vi "WPI_CameraSend Images to PC Loop_EDIT.vi"(8 "error in (no error)":errorcluster, 9 "port":u16, 10 "Image Name":string, 11 "CameraDevRef":T1) -> ()   [LabVIEW 2015]
doc: "This VI is used to send images to the dashboard using the second enet port on the 8 slot controller. This is provided for compatibility, but is higher overhead than using the Camera MJPG approach.\n\nThis software is licensed. Open the labview\\readme\\WPI Robotics Library Open Source License.txt file for more information."
uses:
  <vilib>/Rock Robotics/WPI/Camera/WPI_CameraDevRef.ctl
  <vilib>/Rock Robotics/SystemInterfaces/NetworkCommunication/NetComm_UsageReport_ResourceType.ctl
  <vilib>/Rock Robotics/Network Tables/NT Read Boolean.vi
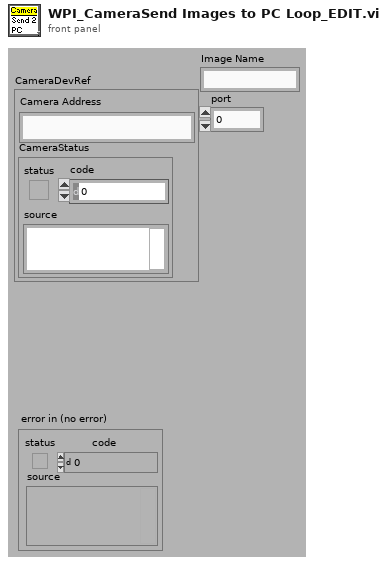
[diagram p1: front panel]
types:
  T1 = typedef "WPI_CameraDevRef.ctl" = cluster{"Camera Address":string, "CameraStatus":errorcluster}
  T2 = cluster{"fps":i32, "compression":i32, "compression 2":i32}
  T3 = typedef "NetComm_UsageReport_ResourceType.ctl" = enum8{"Controller", "Module", "Language", "CANPlugin", "Accelerometer", "ADXL345", "AnalogChannel", "AnalogTrigger", "AnalogTriggerOutput", "CANJaguar", "Compressor", "Counter", "Dashboard", "DigitalInput", "DigitalOutput", "DriverStationCIO", "DriverStationEIO", "DriverStationLCD", "Encoder", "GearTooth", "Gyro", "I2C", "Framework", "Jaguar", "Joystick", "Kinect", "KinectStick", "PIDController", "Preferences", "PWM", "Relay", "RobotDrive", "SerialPort", "Servo", "Solenoid", "SPI", "Task", "Ultrasonic", "Victor", "Button", "Command", "AxisCamera", "PCVideoServer", "SmartDashboard", "Talon", "HiTechnicColorSensor", "HiTechnicAccel", "HiTechnicCompass", "SRF08", "AnalogOutput", "Victor SP", "Talon SRX", "CAN Talon SRX", "ADXL362 Accel", "ADXRS450 Gyro", "Rev SPARK", "Mindsensors SD540", "Digital Filter"}
  T4 = enum16{"Update Mode", "Get Image", "Get Image Data"}
  T5 = typedef "Image Type" = u32
  T6 = typedef "IMAQ Image.ctl" = refnum<image>
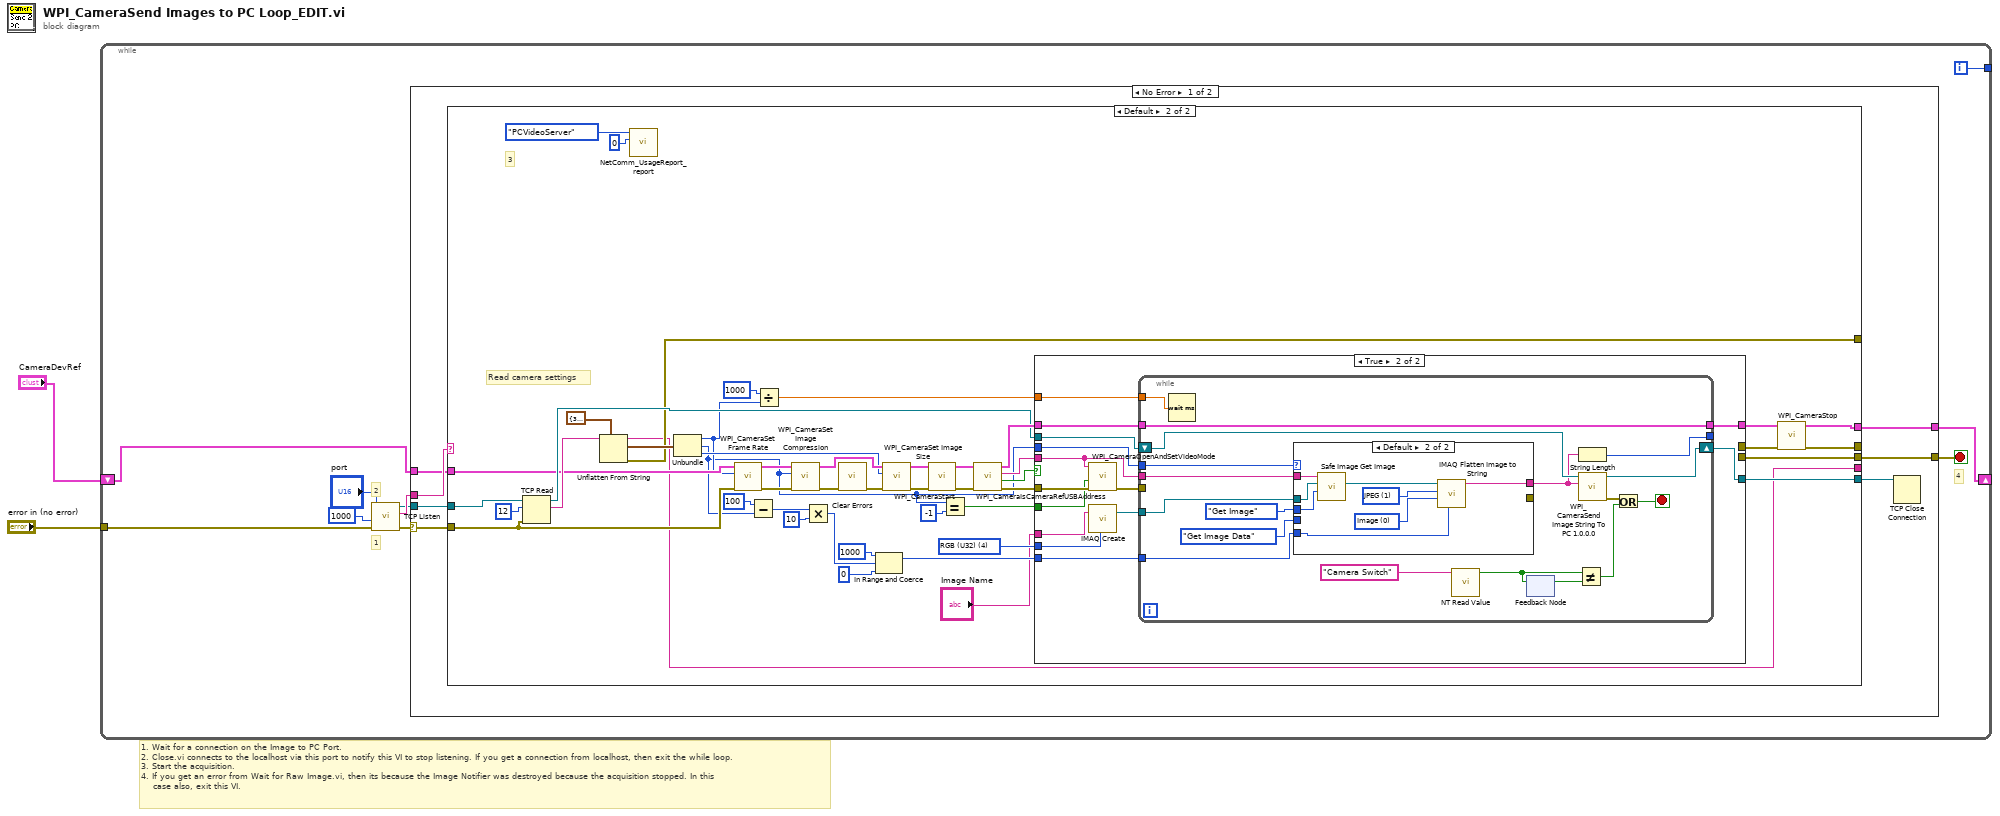
[diagram p0: block diagram]
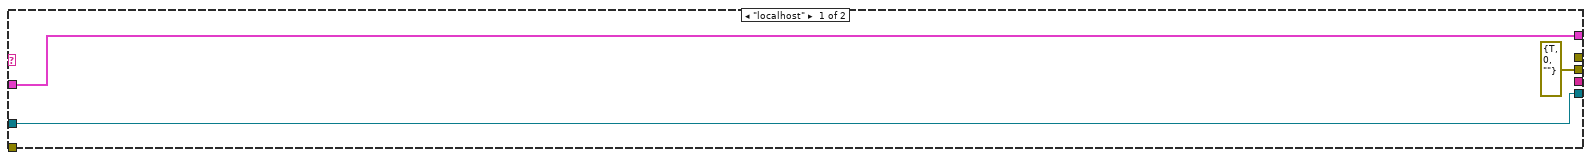
[diagram p2: hidden frame]
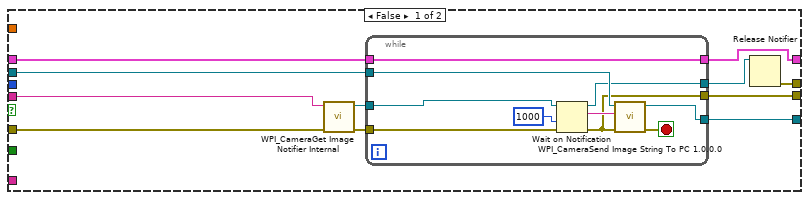
[diagram p3: hidden frame]
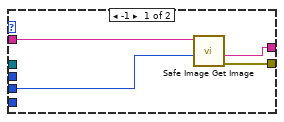
[diagram p4: hidden frame]
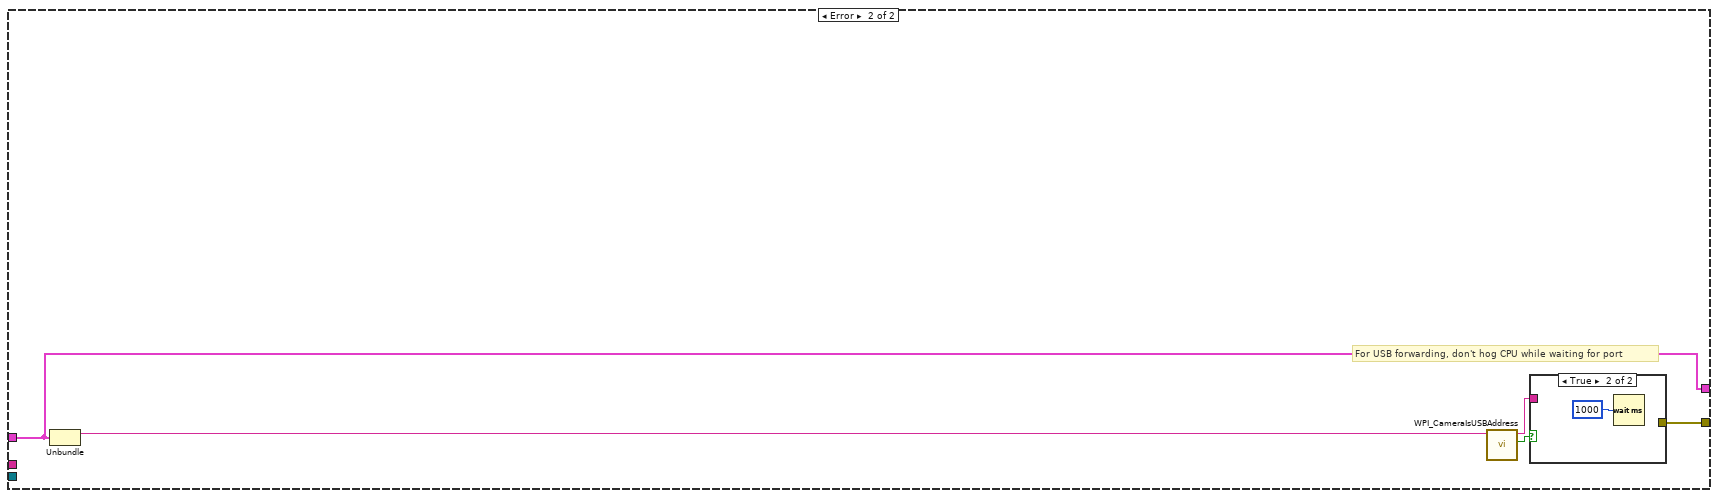
[diagram p5: hidden frame]
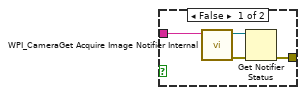
[diagram p6: hidden frame]
diagram:
  # "1. Wait for a connection on the Image to PC Port.\n2. Close.vi connects to the localhost via this port to notify this VI to stop listening. If you get a connection from localhost, then exit the while loop.\n3. Start the acquisition.\n4. If you get an error from Wait for Raw Image.vi, then its because the Image Notifier was destroyed because the acquisition stopped. In this\n    case also, exit this VI."
  n1 = while {
    tunnel: "error in (no error)" -> [w10]
    shift-right: [w12] -> _
    shift-left: "CameraDevRef" -> [w4]
    tunnel: [w5] -> _
    i -> [w5]
    stop <- w8 stop-if-true
    # "4"
    # "1"
    # "2"
    n2 = call <vilib>:"TCP Listen.vi"("error in (no error)"=w10, "timeout ms (wait forever: -1)"=u16 1000 ("port"), "port"="port") -> ("error out"=w7:errorcluster, "remote address"=w11:string, "connection ID"=w9:refnum<k5>)  [unwired: 1 in, 5 out]
    n3 = case shown="No Error" w7 {
      selector: w7 -> [w13 _]
      tunnel: [w19 w138] -> w12
      tunnel: w11 -> [w18 _]
      tunnel: w4 -> [w17 w138]
      tunnel: w9 -> [w16 _]
      tunnel: [w15 w139] -> w8
      frame No Error {
        n4 = case shown="Default" w18 {
          tunnel: [w22 w67] -> w19
          tunnel: w17 -> [w22 w50]
          tunnel: w13 -> [_ w46]
          tunnel: w16 -> [w20 w54]
          tunnel: [errorcluster {"status"=TRUE, "code"=0, "source"=""} ("error out 2") w69] -> w15
          tunnel: [w20 w68] -> w14
          tunnel: [_ w66] -> _
          tunnel: [_ w25] -> _
          tunnel: [_ w24] -> _
          frame "localhost" {
          }
          frame Default {
            w61 = T5 4 items=["Grayscale (U8)", "Grayscale (I16)", "Grayscale (SGL)", "Complex (CSG)", "RGB (U32)", "HSL (U32)", "RGB (U64)", "Grayscale (U16)"] ("Image Type")
            # "Read camera settings"
            # "3"
            n5 = TCP Read(connection ID=w54, bytes to read=12, error in (no error)=w46) -> (connection ID out=w53:refnum<k5>, data out=w51:string)  [unwired: 2 in, 1 out]
            n6 = Unflatten From String(type=T2 {"fps"=30, "compression"=32, "compression 2"=32} ("Camera Settings"), binary string=w51) -> (rest of the binary string=w24:string, value=w43:T2, error out=w25:errorcluster)  [unwired: 3 in]
            n7 = call <vilib>:"NetComm_UsageReport_report.vi"("Instance Number"=u8 0, "Resource Type"=NetComm_UsageReport_ResourceType."PCVideoServer") -> ()  [unwired: 10 in]
            n8 = Unbundle(w43) -> ("fps"=w40:i32, "compression"=w29:i32, "compression 2"=w42:i32)
            n9 = call <vilib>:"WPI_CameraSet Frame Rate.vi"("error in (no error)"=w46, "Frame Rate (fps)"=w40, "CameraDevRef"=w50) -> ("error out"=w45:errorcluster, "CameraDevRef Out"=w49:T1)  [unwired: 7 in]
            n10 = Subtract(x=100, y=w29) -> (x-y=w34:i32)
            n11 = Divide(x=u16 1000 ("port"), y=w40) -> (x/y=w39:dbl)
            n12 = call <vilib>:"WPI_CameraSet Image Compression.vi"("error in (no error)"=w45, "Compression"=w29, "CameraDevRef"=w49) -> ("error out"=w27:errorcluster, "CameraDevRef Out"=w48:T1)  [unwired: 7 in]
            n13 = Multiply(x=w34, y=10) -> (x*y=w36:i32)
            n14 = call <vilib>:"Clear Errors.vi"("error in (no error)"=w27) -> ("error out"=w26:errorcluster)  [unwired: 5 in, 1 out]
            n15 = In Range and Coerce(upper limit=1000, x=w36, lower limit=0) -> (coerced(x)=w32:i32)  [unwired: 1 out]
            n16 = call <vilib>:"WPI_CameraSet Image Size.vi"("error in (no error)"=w26, "Image Size"=w42, "CameraDevRef"=w48) -> ("error out"=w44:errorcluster, "CameraDevRef Out"=w47:T1)  [unwired: 7 in]
            n17 = call <vilib>:"WPI_CameraStart.vi"("error in (no error)"=w44, "CameraDevRef"=w47) -> ("error out"=w58:errorcluster, "CameraDevRef"=w56:T1)  [unwired: 8 out]
            n18 = Equal?(x=w29, y=-1) -> (x = y?=w28:bool)
            n19 = call <vilib>:"WPI_CameraIsCameraRefUSBAddress.vi"("error in (no error)"=w58, "CameraDevRef"=w56) -> ("error out"=w57:errorcluster, "USB?"=w59:bool, "Camera Address Out"=w60:string, "CameraDevRef out"=w55:T1)  [unwired: 6 in]
            n20 = case shown="True" w59 {
              tunnel: w53 -> [w80 w104]
              tunnel: [w79 _] -> w69
              tunnel: [w78 w103] -> w68
              tunnel: w57 -> [w77 w95]
              tunnel: w60 -> [w75 w94]
              tunnel: [w74 w99] -> w65
              tunnel: w55 -> [w73 w100]
              tunnel: [w71 _] -> w64
              tunnel: w61 -> [_ w101]
              tunnel: w32 -> [_ w98]
              tunnel: w39 -> [_ w97]
              tunnel: w29 -> [_ w96]
              tunnel: w28 -> [_ w92]
              tunnel: "Image Name" -> [_ w91]
              frame False {
                n21 = call <vilib>:"WPI_CameraGet Image Notifier Internal.vi"("error in (no error)"=w77, "Camera Address"=w75) -> ("error out"=w76:errorcluster, "Image Notifier"=w72:refnum<notifier>)  [unwired: 8 out]
                n22 = while {
                  tunnel: w76 -> [w86]
                  tunnel: w80 -> [w90]
                  tunnel: [w83] -> w79
                  tunnel: [w88] -> w78
                  tunnel: [w87] -> w74
                  tunnel: w73 -> [w87]
                  tunnel: w72 -> [w85]
                  tunnel: [w81] -> w70
                  stop <- w89 stop-if-true
                  n23 = Wait on Notification(notifier=w85, timeout in ms (-1)=1000 ("Timeout in ms (-1)"), error in (no error)=w86) -> (notifier out=w81:refnum<notifier>, notification=w84:string, error out=w83:errorcluster)  [unwired: 2 out]
                  n24 = call <vilib>:"WPI_CameraSend Image String To PC 1.0.0.0.vi"("error in (no error)"=w83, "String"=w84, "TCP Connection ID"=w90) -> ("error out"=w89:errorcluster, "TCP Connection ID out"=w88:refnum<k5>)  [unwired: 7 out]
                }
                n25 = Release Notifier(notifier=w70) -> (error out=w71:errorcluster)  [unwired: 1 in, 3 out]
              }
              frame True {
                n26 = call <vilib>:"WPI_CameraOpenAndSetVideoMode.vi"("error in (no error)"=w95, "USB JPEG"=w92, "Camera Address Out"=w94) -> ("error out"=w93:errorcluster)  [unwired: 8 in]
                n27 = call "IMAQ Create"("Image Name"=w91, "Image Type"=w101) -> ("New Image"=w102:T6)  [unwired: 3 in, 1 out]
                n28 = while {
                  tunnel: w94 -> [w121]
                  shift-right: [w122] -> w103
                  shift-left: w104 -> [w116]
                  tunnel: w102 -> [w120]
                  tunnel: [w119] -> w99
                  tunnel: w100 -> [w119]
                  tunnel: w98 -> [w118]
                  tunnel: w97 -> [w117]
                  tunnel: [w114] -> _
                  tunnel: w96 -> [w113]
                  tunnel: w93 -> [_]
                  stop <- w106 stop-if-true
                  n29 = Wait (ms)(milliseconds to wait=w117) -> ()  [unwired: 1 out]
                  n30 = case shown="Default" w113 {
                    tunnel: [w125 w134] -> w115
                    tunnel: w121 -> [w126 w130]
                    tunnel: w120 -> [_ w129]
                    tunnel: w118 -> [_ w131]
                    tunnel: [w124 _] -> _
                    tunnel: T4."Get Image Data" ("Operation") -> [w123 _]
                    tunnel: T4."Get Image" ("Operation") -> [_ w127]
                    frame -1 {
                      n31 = call <vilib>:"Safe Image Get Image.vi"("Operation"=w123, "Session In"=w126) -> ("error out"=w124:errorcluster, "Image Data String"=w125:string)  [unwired: 6 in, 2 out]
                    }
                    frame Default {
                      w132 = 0 items=["Image", "Image and Vision Info", "Reference to Image"] ("Type of Flatten (Image and Vision Info)")
                      w133 = 1 items=["None", "JPEG", "PACKED BINARY"] ("Compression (None)")
                      n32 = call <vilib>:"Safe Image Get Image.vi"("Operation"=w127, "Image In"=w129, "Session In"=w130) -> ("Image Out"=w128:T6)  [unwired: 5 in, 3 out]
                      n33 = call "IMAQ Flatten Image to String"("Quality (750)"=w131, "Type of Flatten (Image and Vision Info)"=w132, "Compression (None)"=w133, "Image"=w128) -> ("Data String"=w134:string)  [unwired: 6 in, 1 out]
                    }
                  }
                  n34 = call-poly <vilib>:"NT Read Value.vi"("Name"="Camera Switch") -> ("Boolean"=w109:bool)  [unwired: 9 in, 1 out]
                  n35 = feedback-in #1(w109) -> ()
                  n36 = feedback #1() -> (w108:bool)  [unwired: 1 in]
                  n37 = Not Equal?(x=w109, y=w108) -> (x != y?=w105:bool)
                  n38 = String Length(string=w115) -> (length=w114:i32)
                  n39 = call <vilib>:"WPI_CameraSend Image String To PC 1.0.0.0.vi"("String"=w115, "TCP Connection ID"=w116) -> ("error out"=w107:errorcluster, "TCP Connection ID out"=w122:refnum<k5>)  [unwired: 1 in, 7 out]
                  n40 = Or(x=w107, y=w105) -> (x .or. y?=w106:bool)
                }
              }
            }
            n41 = call <vilib>:"WPI_CameraStop.vi"("error in (no error)"=w64, "CameraDevRef"=w65) -> ("error out"=w66:errorcluster, "CameraDevRef"=w67:T1)  [unwired: 8 out]
          }
        }
        n42 = TCP Close Connection(connection ID=w14) -> ()  [unwired: 1 in, 3 out]
      }
      frame Error {
        # "For USB forwarding, don't hog CPU while waiting for port"
        n43 = Unbundle(w138) -> ("Camera Address"=w137:string)  [unwired: 1 out]
        n44 = call <vilib>:"WPI_CameraIsUSBAddress.vi"("Camera Address In"=w137) -> ("USB?"=w135:bool, "Camera Address Out"=w136:string)  [unwired: 8 in, 1 out]
        n45 = case shown="True" w135 {
          tunnel: [w143 _] -> w139
          tunnel: w136 -> [w140 _]
          frame False {
            n46 = call <vilib>:"WPI_CameraGet Acquire Image Notifier Internal.vi"("Camera Address"=w140) -> ("error out"=w141:errorcluster, "Acquire Image Notifier"=w142:refnum<notifier>)  [unwired: 1 in, 8 out]
            n47 = Get Notifier Status(notifier=w142, error in (no error)=w141) -> (error out=w143:errorcluster)  [unwired: 4 out]
          }
          frame True {
            n48 = Wait (ms)(milliseconds to wait=u32 1000) -> ()  [unwired: 1 out]
          }
        }
      }
    }
  }
